vi "TempConverter.vi"(2 "F temp":dbl, 3 "C temp":dbl) -> (0 "C temp":dbl, 1 "F temp":dbl)   [LabVIEW 2017]
doc: "This VI can transofrm Celsius to Fahrenheit degree and viceversa"
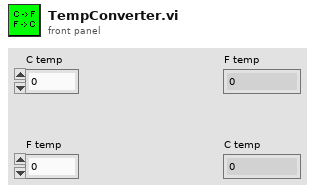
[diagram p1: front panel]
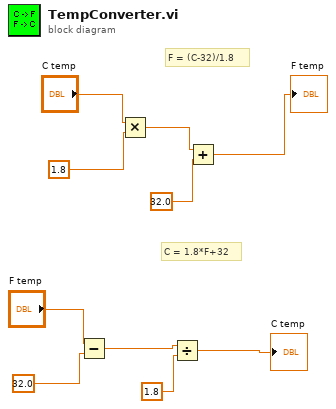
[diagram p0: block diagram]
diagram:
  # "C = 1.8*F+32"
  # "F = (C-32)/1.8"
  n1 = Subtract(x="F temp", y=32.0) -> (x-y=w4:dbl)
  n2 = Multiply(x="C temp", y=1.8) -> (x*y=w8:dbl)
  n3 = Divide(x=w4, y=1.8) -> (x/y=→"C temp":dbl)
  n4 = Add(x=w8, y=32.0) -> (x+y=→"F temp":dbl)
